vi "gentec-M-Link.get Energy.vi"(1 "ADC Counts":u16, 2 "Range":T1 items=["1f", "3f", "10f", "30f", "100f", "300f", "1p", "3p", "10p", "30p", "100p", "300p", "1n", "3n", "10n", "30n", "100n", "300n", "1u", "3u", "10u", "30u", "100u", "300u", "1m", "3m", "10m", "30m", "100m", "300m", "1", "3", "10", "30", "100", "300", "1K", "3K", "10K", "30K", "100K", "300K", "1M", "3M", "10M", "30M", "100M", "300M"]) -> (0 "Energy [J]":dbl format="%#_6p")   [LabVIEW 2014, in "gentec-M-Link - Driver.lvlib"]
doc: "This VI calculates the Energy in J depending on the ADC Counts and the current Range."
uses:
  gentec-M-Link - Driver.lvlib
  Type Defs/gentec-M-Link.Range.ctl
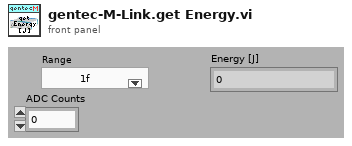
[diagram p1: front panel]
types:
  T1 = typedef "gentec-M-Link - Driver.lvlib/gentec-M-Link.Range.ctl" = u16
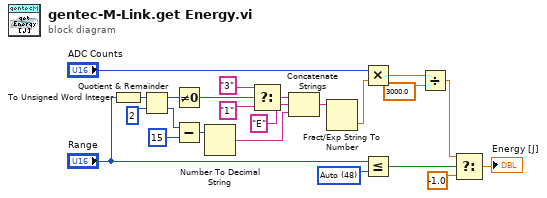
[diagram p0: block diagram]
diagram:
  w21 = T1 48 items=["1f", "3f", "10f", "30f", "100f", "300f", "1p", "3p", "10p", "30p", "100p", "300p", "1n", "3n", "10n", "30n", "100n", "300n", "1u", "3u", "10u", "30u", "100u", "300u", "1m", "3m", "10m", "30m", "100m", "300m", "1", "3", "10", "30", "100", "300", "1K", "3K", "10K", "30K", "100K", "300K", "1M", "3M", "10M", "30M", "100M", "300M", "Auto"] ("y")
  n1 = To Unsigned Word Integer(number="Range") -> (unsigned 16bit integer=w16:T1)
  n2 = Quotient & Remainder(x=w16, y=2) -> (x-y*floor(x/y)=w14:i32, floor(x/y)=w8:i32)
  n3 = Not Equal To 0?(x=w14) -> (x != 0?=w13:bool)
  n4 = Subtract(x=w8, y=15) -> (x-y=w6:i32)
  n5 = Number To Decimal String(number=w6) -> (decimal integer string=w5:string)  [unwired: 1 in]
  n6 = Select(t="3", s=w13, f="1") -> (s? t:f=w10:string)
  n7 = Concatenate Strings(w10, "E" ("string"), w5) -> (w4:string)
  n8 = Fract/Exp String To Number(string=w4) -> (number=w2:dbl)  [unwired: 3 in, 1 out]
  n9 = Multiply(x="ADC Counts", y=w2) -> (x*y=w23:dbl)
  n10 = Less Or Equal?(x="Range", y=w21) -> (x <= y?=w20:bool)
  n11 = Divide(x=w23, y=3000.0) -> (x/y=w17:dbl)
  n12 = Select(t=w17, s=w20, f=-1.0) -> (s? t:f=→"Energy [J]":dbl)
